vi "Init_DM_DUAL_V2.vi"(7 "BM Flat":bool, 8 "BM Flat File":string[](array[string]), 9 "Mirror Modes File":string, 10 "DM Mapping File":string, 11 "Base File Path":path) -> (3 "reference out":refnum<k7>)   [LabVIEW 2016]
uses:
  Hardware Configuration/Hardware Configuration Controls/Standard Action.ctl
  <vilib>/Utility/file.llb/Read From Spreadsheet File (DBL).vi
  <vilib>/Utility/file.llb/Read From Spreadsheet File (string).vi
panel:
  out "IDs":i32[](array[numeric])
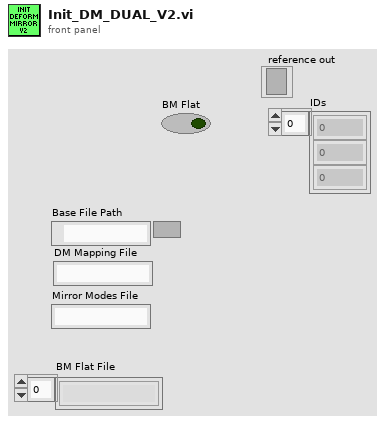
[diagram p1: front panel]
types:
  T1 = typedef "Standard Action.ctl" = enum16{"Read", "Write"}
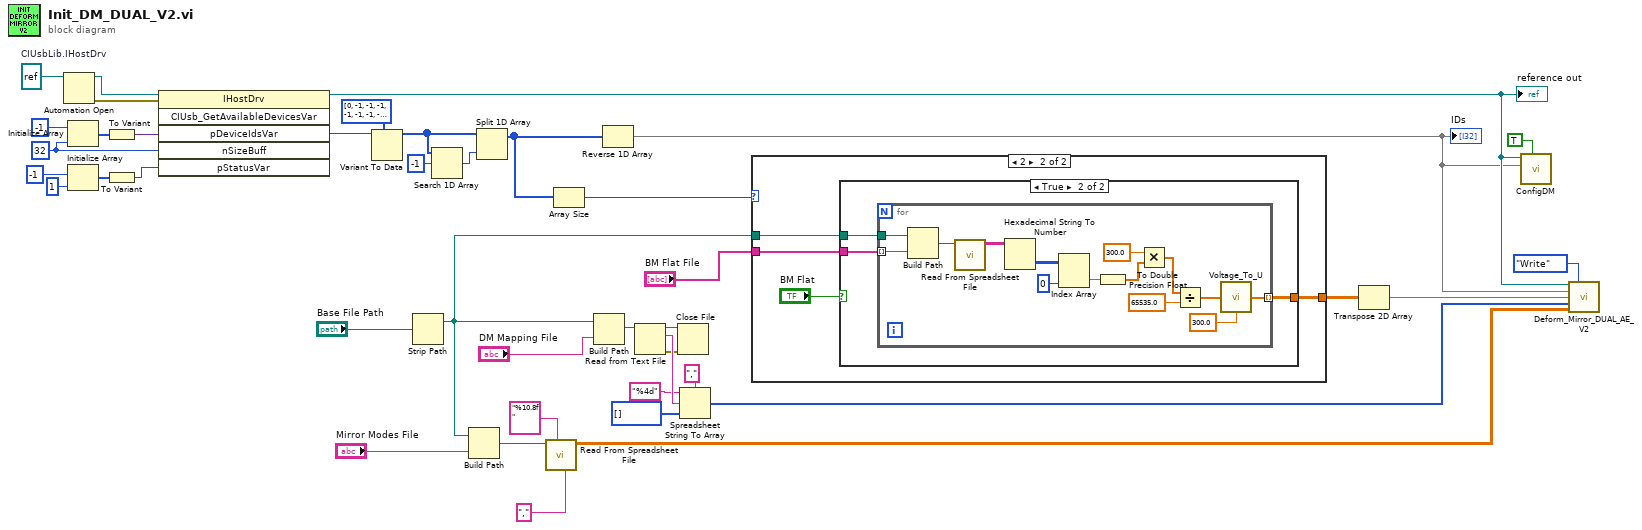
[diagram p0: block diagram]
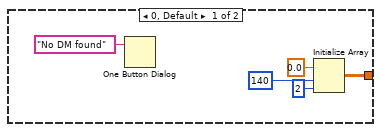
[diagram p2: hidden frame]
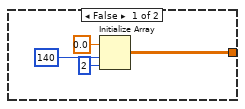
[diagram p3: hidden frame]
diagram:
  w36 = 32 ("dimension size")
  w27 = refnum<k7> refnum  # CIUsbLib.IHostDrv
  n1 = Automation Open(Automation Refnum=w27) -> (Automation Refnum=w32:refnum<k7>, error out=w33:errorcluster)  [unwired: 1 in, 2 out]
  n2 = Initialize Array(-1 ("element"), w36) -> (w29:i32[])
  n3 = Initialize Array(-1 ("element"), 1 ("dimension size")) -> (w28:i32[])
  n4 = To Variant(anything=w29) -> (Variant=w30:variant)
  n5 = To Variant(anything=w28) -> (Variant=w35:variant)
  n6 = invoke class="IHostDrv" method="CIUsb_GetAvailableDevicesVar"(reference=w32, error in=w33, "pDeviceIdsVar"=w30, "nSizeBuff"=w36, "pStatusVar"=w35) -> (reference out=w13:refnum<k7>, "pDeviceIdsVar"=w41:variant)  [unwired: 1 in, 4 out]
  "reference out" <- w13
  n7 = Variant To Data(type=i32[] [0, -1, -1, -1, -1, -1, -1, -1, -1, -1, -1, -1, -1, -1, -1, -1, -1, -1, -1, -1, -1, -1, -1, -1, -1, -1, -1, -1, -1, -1, -1, -1] ("pDeviceIDs"), Variant=w41) -> (data=w39:i32[])  [unwired: 1 in, 1 out]
  n8 = Strip Path(path="Base File Path") -> (stripped path=w17:path)  [unwired: 1 out]
  n9 = Search 1D Array(1D array=w39, element=-1) -> (index of element=w38:i32)  [unwired: 1 in]
  n10 = Build Path(base path=w17, name or relative path="Mirror Modes File") -> (appended path=w18:path)
  n11 = Split 1D Array(array=w39, index=w38) -> (first subarray=w3:i32[])  [unwired: 1 out]
  n12 = call-poly <vilib>:"Read From Spreadsheet File.vi"("delimiter (\\t)"="," ("delimiter (\\t)"), "format (%.3f)"="%10.8f", "file path (dialog if empty)"=w18) -> ("all rows"=w8:dbl[][])  [unwired: 2 in, 6 out]
  n13 = Array Size(array=w3) -> (size(s)=w15:i32)
  n14 = Build Path(base path=w17, name or relative path="DM Mapping File") -> (appended path=w20:path)
  n15 = Reverse 1D Array(array=w3) -> (reversed array=w1:i32[])
  "IDs" <- w1
  n16 = Read from Text File(file (use dialog)=w20) -> (refnum out=w22:refnum<file>, text=w26:string, error out=w21:errorcluster)  [unwired: 1 in, 3 out]
  n17 = Close File(refnum=w22, error in=w21) -> ()  [unwired: 2 out]
  n18 = Spreadsheet String To Array(delimiter (Tab)=",", format string="%4d", spreadsheet string=w26, array type (2D Dbl)=i32[] []) -> (array=w5:i32[])
  n19 = case shown="2" w15 {
    tunnel: w17 -> [_ w50]
    tunnel: "BM Flat File" -> [_ w49]
    tunnel: [w42 w48] -> w4
    frame 0, Default {
      n20 = One Button Dialog(message="No DM found") -> ()  [unwired: 1 in, 1 out]
      n21 = Initialize Array(0.0 ("element"), 140 ("dimension size"), 2 ("dimension size")) -> (w42:dbl[][])
    }
    frame 2 {
      n22 = case shown="True" "BM Flat" {
        tunnel: w50 -> [_ w57]
        tunnel: w49 -> [_ w55]
        tunnel: [w51 w56] -> w48
        frame False {
          n23 = Initialize Array(0.0 ("element"), 140 ("dimension size"), 2 ("dimension size")) -> (w51:dbl[][])
        }
        frame True {
          n24 = for {
            tunnel: w57 -> [w71]
            tunnel: [w58] -> w56 mode=indexing
            tunnel: w55 -> [w61] mode=indexing
            n25 = Build Path(base path=w71, name or relative path=w61) -> (appended path=w70:path)
            n26 = call-poly <vilib>:"Read From Spreadsheet File.vi"("file path (dialog if empty)"=w70) -> ("all rows"=w69:string[][])  [unwired: 3 in, 7 out]
            n27 = Hexadecimal String To Number(string=w69) -> (number=w68:u32[][])  [unwired: 2 in, 1 out]
            n28 = Index Array(array=w68, index (col)=0 ("disabled index (col)")) -> (element=w66:u32[])  [unwired: 1 in]
            n29 = To Double Precision Float(number=w66) -> (double precision float=w62:dbl[])
            n30 = Multiply(x=300.0 ("y"), y=w62) -> (x*y=w65:dbl[])
            n31 = Divide(x=w65, y=65535.0) -> (x/y=w59:dbl[])
            n32 = call "Voltage_To_U.vi"("Voltages In (Volts)"=w59, "Mirror Max Voltage (Volts)"=300.0) -> ("Pixel Value (-1 to 1)"=w58:dbl[])  [unwired: 13 in]
          }
        }
      }
    }
  }
  n33 = Transpose 2D Array(2D array=w4) -> (transposed array=w2:dbl[][])
  n34 = call "ConfigDM.vi"("High Voltage"=TRUE, "Dev IDs"=w1, "Automation Refnum in"=w13) -> ()  [unwired: 7 in, 2 out]
  n35 = call "Deform_Mirror_DUAL_AE_V2.vi"("Refnum In"=w13, "Action"=Standard_Action."Write", "IDs In"=w1, "Flat Files In"=w2, "Multi Map Data In"=w5, "Mode Matrix"=w8) -> ()  [unwired: 5 in, 5 out]
